vi "Example.vi"() -> ()   [LabVIEW 2019]
panel:
  out "x+y":dbl
  in  "x":dbl
  in  "y":dbl
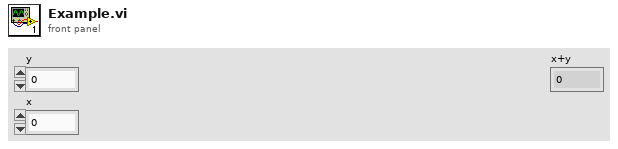
[diagram p1: front panel]
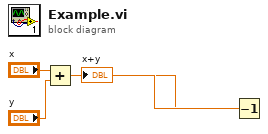
[diagram p0: block diagram]
diagram:
  n1 = Add(x="x", y="y") -> (x+y=w2:dbl)
  n2 = Decrement(x=w2) -> (x-1=→"x+y":dbl)
